vi "GetProjectConditionalDeactivationValueByKey.vi"(7 "Value":string, 8 "Fehler (Eingang, kein Fehler)":errorcluster, 9 "Values":string[](array[string]), 10 "Keys":string[](array[string]), 11 "Key":string) -> (0 "Fehler (Ausgang)":errorcluster, 1 "Values out":string[](array[string]), 2 "Keys out":string[](array[string]), 3 "Value out":string, 4 "Value matched":bool)   [LabVIEW 2015, in "ConditionalDeactivation.lvlib"]
uses:
  ConditionalDeactivation.lvlib
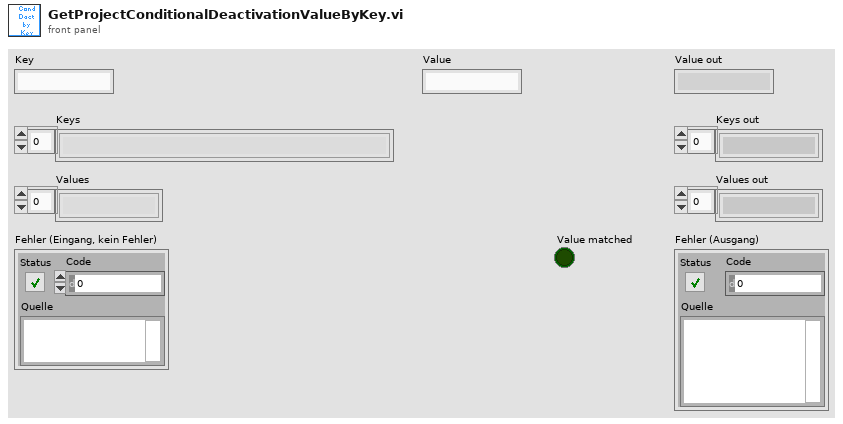
[diagram p1: front panel]
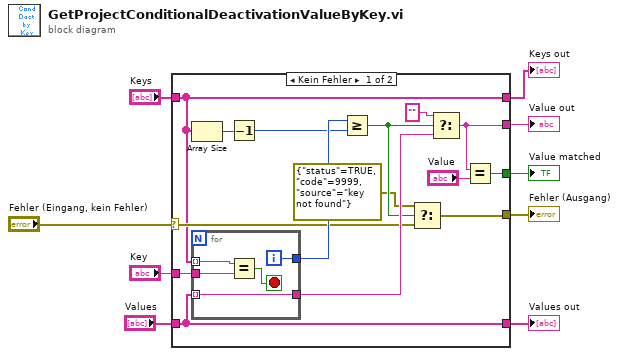
[diagram p0: block diagram]
diagram:
  n1 = case shown="Kein Fehler" "Fehler (Eingang, kein Fehler)" {
    selector: "Fehler (Eingang, kein Fehler)" -> [w16 w32]
    tunnel: [w11 _] -> w9
    tunnel: [w17 w32] -> w8
    tunnel: "Values" -> [w14 w31]
    tunnel: "Keys" -> [w13 w30]
    tunnel: [w14 w31] -> w4
    tunnel: [w13 w30] -> w3
    tunnel: "Key" -> [w15 _]
    tunnel: [w10 _] -> w1
    frame No Error {
      n2 = Array Size(array=w13) -> (size(s)=w23:i32)
      n3 = for {
        tunnel: w13 -> [w29] mode=indexing
        tunnel: w14 -> [w26] mode=indexing
        tunnel: w15 -> [w28]
        tunnel: [w26] -> w22
        tunnel: [w25] -> w24
        i -> [w25]
        stop <- w27 stop-if-true
        n4 = Equal?(x=w29, y=w28) -> (x = y?=w27:bool)
      }
      n5 = Decrement(x=w23) -> (x-1=w20:i32)
      n6 = Greater Or Equal?(x=w24, y=w20) -> (x >= y?=w19:bool)
      n7 = Select(t=errorcluster {"status"=TRUE, "code"=9999, "source"="key not found"} ("Fehlerkonstante"), s=w19, f=w16) -> (s? t:f=w17:errorcluster)
      n8 = Select(t="", s=w19, f=w22) -> (s? t:f=w11:string)
      n9 = Equal?(x=w11, y="Value") -> (x = y?=w10:bool)
    }
    frame Error {
    }
  }
  "Fehler (Ausgang)" <- w8
  "Value out" <- w9
  "Values out" <- w4
  "Keys out" <- w3
  "Value matched" <- w1
